vi "niRFUtil RFHS Channelizer ChannelizerRef CSG phaseII.vi"(0 "Channelizer Ref":refnum<data-value>, 1 "Reset":bool, 2 "Benchmark Task":T1, 5 "Source Channelizer Ref":refnum<data-value>, 7 "Length":i32=-1, 9 "Channnel":i32, 11 "error in (no error)":errorcluster, 13 "CPU Context":string) -> (4 "Channelizer Ref (out)":refnum<data-value>, 6 "Channel Data":csg[](array[numeric]), 8 "Channel Data Len":u32[](array[numeric]), 15 "error out":errorcluster)   [LabVIEW 2015, in "niRFUtil.lvlib"]
uses:
  niRFUtil.lvlib
  Utilities/Benchmark/niRFUtil RFHS Benchmark Task.ctl
  Includes/niRFUtil RFHS Channelizer ChannelizerInfo CSG.ctl
  Includes/niRFUtil RFHS Channelizer FilterRef.ctl
  Includes/niRFUtil RFHS Channelizer ChannelizerBufferingMode.ctl
  Utilities/Data FIFO/niRFUtil RFHS FIFO Reference.ctl
  Utilities/Data FIFO/niRFUtil RFHS FIFO.ctl
  Includes/niRFUtil RFHS Channelizer ChannelizerType.ctl
  Includes/niRFUtil RFHS Channelizer ChannelizerFlags.ctl
  Includes/niRFUtil RFHS Channelizer ChannelizerErrors.ctl
  Utilities/niRFUtil RFHS Util Data Subset.ctl
  niRFUtil RFHS Channelizer AdjustDataSubsetSpecification.vi
  niRFUtil RFHS Channelizer BufferLen CSG.vi
  niRFUtil RFHS Channelizer ChannelizerHandleDllError.vi
  Utilities/niRFUtil RFHS Util Process CPU Context.vi
  niRFUtil RFHS Channelizer ProcessCPUContext.vi
  Utilities/niRFUtil RFHS Util Dll Path.vi
panel:
  out "Time":u32
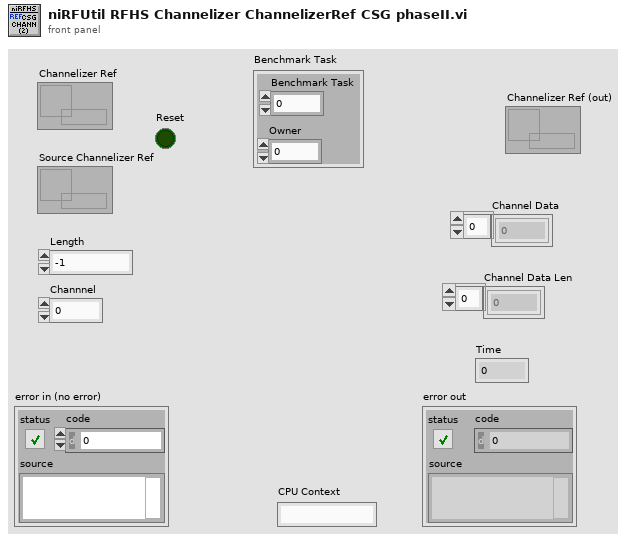
[diagram p1: front panel]
types:
  T1 = typedef "niRFUtil.lvlib/niRFUtil RFHS Benchmark Task.ctl" = cluster{"Benchmark Task":u64, "Owner":u32}
  T2 = typedef "niRFUtil.lvlib/niRFUtil RFHS Channelizer ChannelizerErrors.ctl" = enum32{"No Error", "Invalid Channel", "Internal Error", "Invalid Channel fs", "Invalid Phase Shift", "Invalid fs", "Invalid Number Of Channles", "Invalid FFT Channel fs", "Invalid Resampler Channel fs", "Not a 15kHz Multiple", "Invalid Channel fc", "Invalid passBW/stopBW", "Coerced Rejection", "Requires Internal Buffer", "Duplicated Destination Channel Name", "Configuration Format Error", "Illegal Execution state", "DLL not found", "DLL loading failure", "AVX instruction failure"}
  T3 = typedef "niRFUtil.lvlib/niRFUtil RFHS Util Data Subset.ctl" = cluster{"Offset":i32, "Length":i32}
  T4 = typedef "niRFUtil.lvlib/niRFUtil RFHS Channelizer ChannelizerInfo CSG.ctl" = cluster{"Filter LVRef":T5, "Mode":T6, "History":csg[], "Buffer":csg[], "FIFO":T7, "History Len":u32, "Float Cache":csg[], "Double Cache":cdb[], "Type":T9, "Resample Phase":dbl, "fft1Descriptors":u64[], "fft2Descriptors":u64[], "FFT tBuf":csg[], "guardBandLen":i32, "FFT History":csg[], "FFT History Len":u32, "FFTInitDone":u32, "FFT Filter LVRefs":T5[], "FFT fc Offs":u32[], "fft2Sizes":u32[], "BufferW":u32[], "BufferR":u32[], "Buff Off":u32[], "Phase0 (fshift)":dbl[], "Phase (fshift)":dbl[], "fs phase step":dbl[], "Resample Step":dbl, "Flags":T10, "Reset Cnt":i64, "Filter Pass":u32, "Stages":variant[]}
  T5 = typedef "niRFUtil.lvlib/niRFUtil RFHS Channelizer FilterRef.ctl" = cluster{"Ref":u64, "GUID":u64, "Upsample":i32, "Downsample":i32, "Size":i32, "Num Taps":i32}
  T6 = typedef "niRFUtil.lvlib/niRFUtil RFHS Channelizer ChannelizerBufferingMode.ctl" = enum32{"Unbuffered", "Finite", "Continuous"}
  T7 = typedef "niRFUtil.lvlib/niRFUtil RFHS FIFO Reference.ctl" = cluster{"Read Lock":refnum<data-value>, "Info":T8, "Write Lock":refnum<data-value>}
  T8 = typedef "niRFUtil.lvlib/niRFUtil RFHS FIFO.ctl" = cluster{"ID":u64, "Length":u32}
  T9 = typedef "niRFUtil.lvlib/niRFUtil RFHS Channelizer ChannelizerType.ctl" = enum32{"Auto", "Frequency Shift Only", "Resampler Only"}
  T10 = typedef "niRFUtil.lvlib/niRFUtil RFHS Channelizer ChannelizerFlags.ctl" = u32
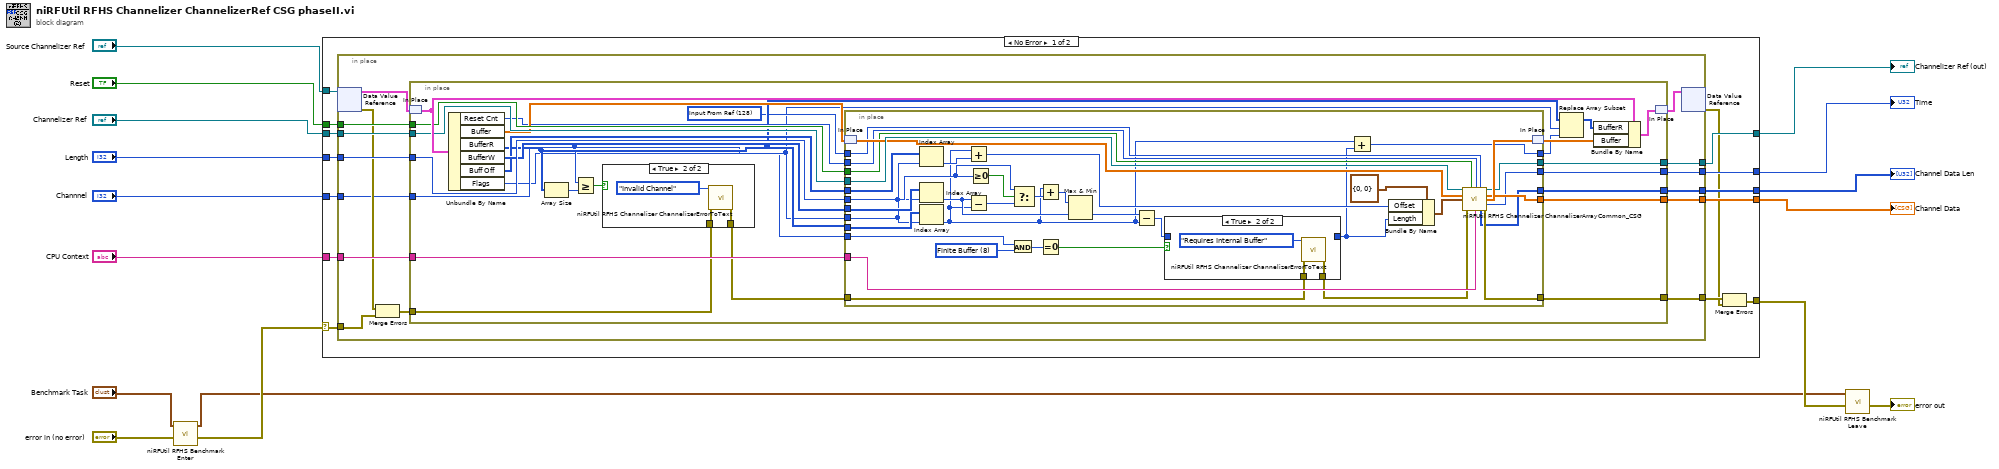
[diagram p0: block diagram]
diagram:
  n1 = call "niRFUtil RFHS Benchmark Enter.vi"("error in (no error)"="error in (no error)", "Benchmark Task (Parent)"="Benchmark Task") -> ("error out"=w13:errorcluster, "Benchmark Task (Self)"=w5:T1)  [unwired: 8 in]
  n2 = case shown="No Error" w13 {
    selector: w13 -> [w30 w119]
    tunnel: "Reset" -> [w29 _]
    tunnel: [w17 w119] -> w14
    tunnel: [w28 _] -> w10
    tunnel: [w27 _] -> w9
    tunnel: "CPU Context" -> [w26 _]
    tunnel: "Channelizer Ref" -> [w25 w118]
    tunnel: [w24 w118] -> w6
    tunnel: "Source Channelizer Ref" -> [w23 _]
    tunnel: "Length" -> [w22 _]
    tunnel: [w21 _] -> w2
    tunnel: "Channnel" -> [w20 _]
    frame No Error {
      n3 = in-place {
        in-place-border: w30 -> [w33]
        in-place-border: w29 -> [w39]
        in-place-border: [w41] -> w19
        in-place-border: [w42] -> w28
        in-place-border: [w43] -> w27
        in-place-border: w26 -> [w40]
        in-place-border: w25 -> [w45]
        in-place-border: [w44] -> w24
        in-place-border: w22 -> [w38]
        in-place-border: [w35] -> w21
        in-place-border: w20 -> [w31]
        n4 = in-place-dvr #1(w23) -> (w37:T4, w34:errorcluster)
        n5 = Merge Errors(w34, w33) -> (w32:errorcluster)
        n6 = in-place {
          in-place-border: w45 -> [w66]
          in-place-border: w32 -> [w50]
          in-place-border: [w61] -> w44
          in-place-border: [w62] -> w43
          in-place-border: [w63] -> w42
          in-place-border: [w64] -> w41
          in-place-border: w40 -> [w67]
          in-place-border: w39 -> [w65]
          in-place-border: w38 -> [w71]
          in-place-border: [w55] -> w35
          in-place-border: w31 -> [w47]
          w48 = T10 128 items=["None"=0, "Skip Stage 1"=1, "FFT Stage"=2, "Frequency Shift"=4, "Finite Buffer"=8, "Reset"=16, "Input Len Estimate"=32, "C buffers"=64, "Input From Ref"=128] ("Flags")
          n7 = in-place-match #2(w37) -> (w69:T4)
          n8 = Unbundle By Name(w69) -> ("Reset Cnt"=w56:i64, "Buffer"=w59:csg[], "BufferR"=w53:u32[], "BufferW"=w70:u32[], "Buff Off"=w54:u32[], "Flags"=w46:T10)
          n9 = Array Size(array=w53) -> (size(s)=w52:i32)
          n10 = Greater Or Equal?(x=w47, y=w52) -> (x >= y?=w51:bool)
          n11 = case shown="True" w51 {
            tunnel: w50 -> [w72 w74]
            tunnel: [w72 w73] -> w49
            frame False {
            }
            frame True {
              n12 = call "niRFUtil RFHS Channelizer ChannelizerErrorToText.vi"("Error List"=niRFUtil_RFHS_Channelizer_ChannelizerErrors."Invalid Channel", "error in (no error)"=w74) -> ("error out"=w73:errorcluster)  [unwired: 13 in]
            }
          }
          n13 = in-place {
            in-place-border: w71 -> [w109]
            in-place-border: w70 -> [w104]
            in-place-border: w53 -> [w105]
            in-place-border: [w83] -> w57
            in-place-border: w49 -> [w80]
            in-place-border: w67 -> [w94]
            in-place-border: w66 -> [w97]
            in-place-border: w65 -> [w93]
            in-place-border: [w98] -> w64
            in-place-border: [w100] -> w63
            in-place-border: [w99] -> w62
            in-place-border: [w101] -> w61
            in-place-border: w56 -> [w92]
            in-place-border: [w91] -> w55
            in-place-border: w54 -> [w90]
            in-place-border: w47 -> [w87]
            in-place-border: w48 -> [w86]
            in-place-border: w46 -> [w79]
            w82 = T10 8 items=["None"=0, "Skip Stage 1"=1, "FFT Stage"=2, "Frequency Shift"=4, "Finite Buffer"=8, "Reset"=16, "Input Len Estimate"=32, "C buffers"=64, "Input From Ref"=128] ("y")
            n14 = in-place-match #3(w59) -> (w95:csg[])
            n15 = Index Array(array=w90, index=w87) -> (element=w89:u32)
            n16 = Index Array(array=w104, index=w87) -> (element=w103:u32)
            n17 = Index Array(array=w105, index=w87) -> (element=w77:u32)
            n18 = Add(x=w77, y=w89) -> (x+y=w88:u32)
            n19 = Subtract(x=w103, y=w77) -> (x-y=w108:u32)
            n20 = Greater Or Equal To 0?(x=w109) -> (x >= 0?=w110:bool)
            n21 = And(x=w79, y=w82) -> (x .and. y?=w81:T10)
            n22 = Select(t=w109, s=w110, f=w108) -> (s? t:f=w107:u32)
            n23 = Add(x=w77, y=w107) -> (x+y=w111:u32)
            n24 = Equal To 0?(x=w81) -> (x = 0?=w78:bool)
            n25 = Max & Min(x=w111, y=w103) -> (min(x,y)=w106:u32)  [unwired: 1 out]
            n26 = Subtract(x=w106, y=w77) -> (x-y=w84:u32)
            n27 = case shown="True" w78 {
              tunnel: w80 -> [w114 w116]
              tunnel: [w114 w115] -> w85
              tunnel: [w113 _] -> w76
              tunnel: w84 -> [w113 _]
              frame False {
              }
              frame True {
                n28 = call "niRFUtil RFHS Channelizer ChannelizerErrorToText.vi"("Error List"=niRFUtil_RFHS_Channelizer_ChannelizerErrors."Requires Internal Buffer", "error in (no error)"=w116) -> ("error out"=w115:errorcluster)  [unwired: 13 in]
              }
            }
            n29 = Add(x=w77, y=w76) -> (x+y=w83:u32)
            n30 = Bundle By Name(cluster=T3 {"Offset"=0, "Length"=0} ("Data Subset"), "Offset"=w88, "Length"=w76) -> (w96:T3)
            n31 = call "niRFUtil RFHS Channelizer ChannelizerArrayCommon_CSG.vi"("Channelizer Ref"=w97, "Reset"=w93, "Reset Cnt"=w92, "Caller Flags"=w86, "Data"=w95, "Data Subset"=w96, "error in (no error)"=w85, "CPU Context"=w94) -> ("Channelizer Ref (out)"=w101:refnum<data-value>, "Channel Data"=w100:csg[], "Data (out)"=w102:csg[], "Time"=w99:u32, "Channel Data Len"=w91:u32[], "error out"=w98:errorcluster)  [unwired: 2 in]
            n32 = in-place-match #3(w102) -> (w60:csg[])
          }
          n33 = Replace Array Subset(array=w53, new element=w57, index=w47) -> (w58:u32[])
          n34 = Bundle By Name(cluster=w69, "BufferR"=w58, "Buffer"=w60) -> (w68:T4)
          n35 = in-place-match #2(w68) -> (w36:T4)
        }
        n36 = in-place-dvr #1(w36) -> (w18:errorcluster)  [unwired: 1 out]
      }
      n37 = Merge Errors(w19, w18) -> (w17:errorcluster)
    }
    frame Error {
    }
  }
  "Channel Data" <- w10
  "Time" <- w9
  "Channelizer Ref (out)" <- w6
  "Channel Data Len" <- w2
  n38 = call "niRFUtil RFHS Benchmark Leave.vi"("error in (no error)"=w14, "Benchmark Task Self"=w5) -> ("error out"=→"error out":errorcluster)  [unwired: 8 in, 1 out]
